vi "DAQ_E_mIO_DIO.get input port.vi"(0 "i ref in":refnum<vi>, 5 "error in (no error)":errorcluster) -> (14 "i ref out":refnum<vi>, 16 "portList":tag="Dev1/port0", 19 "error out":errorcluster)   [LabVIEW 2014, in "DAQ_E_mIO_DIO.lvlib"]
doc: "Gets the name of the port for digital input.\n\nLicense Agreement for the BaseProcess class:\n\nCopyright (C)\nGesellschaft für Schwerionenforschung, GSI\nPlanckstr. 1\n64291 Darmstadt\nGermany\n\nContact: D.Beck@gsi.de \n\nThis program is free software; you can redistribute it and/or modify it under the terms of the \nGNU General Public License as published by the Free Software Foundation; either version 2 of the license, or (at your option) any later version.\n\nThis program is distributed in the hope that it will be useful, but WITHOUT ANY WARRANTY; without even the implied warranty of MERCHANTABILITY or FITNESS FOR A PARTICULAR PURPOSE. See the GNU General License for more details (http://www.gnu.org).\n\nGesellschaft für Schwerionenforschung, GSI\nPlanckstr. 1, 64291 Darmstadt, Germany\nFor all questions and ideas contact: M.Richter@gsi.de, H.Brand@gsi.de or D.Beck@gsi.de.\nLast update: 25-SEP-2002"
uses:
  DAQ_E_mIO_DIO.lvlib
  CSCore/BaseProcess/BaseProcess.lvlib
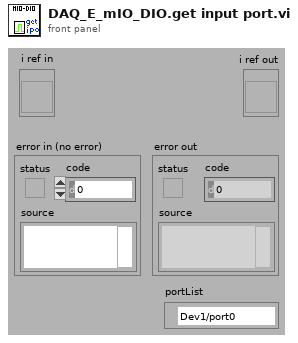
[diagram p1: front panel]
types:
  T1 = typedef "BaseProcess.lvlib/BaseProcess.i attribute.ctl" = cluster{"EventStatus":string, "EventError":i32, "PresetEvtWatchD":i32, "PresetPdcWatchD":i32, "EventTimeout":i32, "PeriodicInterval":i32, "Interface":string[], "Address":string[], "Special":string[], "PeriodicError":i32, "PeriodicStatus":string, "SuperProc":string, "Descriptors":T2[], "CaseRef":refnum<vi>, "PdcRef":refnum<vi>, "Thread Ref":refnum<vi>, "eventErrorID":i32, "eventStatusID":i32, "periodicErrorID":i32, "periodicStatusID":i32, "pdcCtrID":i32}
  T2 = typedef "BaseProcess.lvlib/BaseProcess.descriptor definition.ctl" = cluster{"selector":string, "descriptor":T3}
  T3 = typedef "BaseProcess.lvlib/BaseProcess.descriptor string definition.ctl" = string
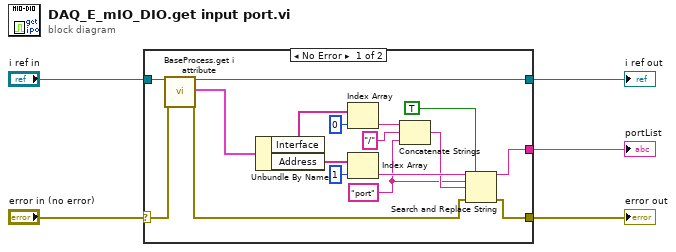
[diagram p0: block diagram]
diagram:
  n1 = case shown="No Error" "error in (no error)" {
    selector: "error in (no error)" -> [w15 w23]
    tunnel: [w22 w24] -> w1
    tunnel: [w8 w23] -> w3
    tunnel: "i ref in" -> [w21 w24]
    tunnel: [w6 _] -> w2
    frame No Error {
      w10 = "port" ("search string")
      n2 = call "BaseProcess.get i attribute.vi"("i ref in"=w21, "error in (no error)"=w15) -> ("i ref out"=w22:refnum<vi>, "i attribute"=w16:T1, "error out"=w9:errorcluster)  [unwired: 15 in]
      n3 = Unbundle By Name(w16) -> ("Interface"=w17:string[], "Address"=w19:string[])
      n4 = Index Array(array=w17, index=0) -> (element=w13:string)
      n5 = Index Array(array=w19, index=1) -> (element=w14:string)
      n6 = Concatenate Strings(w13, "/" ("string"), w10) -> (w11:string)
      n7 = Search and Replace String(replace all?=TRUE ("replace all? (F)"), input string=w14, search string=w10, replace string=w11, error in=w9) -> (result string=w6:string, error out=w8:errorcluster)  [unwired: 3 in, 2 out]
    }
    frame Error {
    }
  }
  "error out" <- w3
  "i ref out" <- w1
  "portList" <- w2
